vi "Demo - Log Analog and Digital Inputs to CSV File.vi"() -> ()   [LabVIEW 2021]
uses:
  TypeDefs/Enum - Machine State.ctl
  TypeDefs/TypeDef - Cluster of DAQiFi Device Properties.ctl
  TypeDefs/Enum - Connection Type.ctl
  <vilib>/Utility/file.llb/Write Delimited Spreadsheet (DBL).vi
  <vilib>/ErrorRing/Error Ring.xnode
panel:
  out "Digital Inputs":T1(graph)
  in  "Path - Saved CSV File":path=path "C:/Daqifi datafile.CSV"
  in  "Sampling Rate (Hz)":i32=1 min=1 max=1000 step=1
  out "Program Status":string
  in  "Stop":bool
  out "Analog Inputs":T2(graph)
  in  "DAQ IP Address or COM Port":string="192.168.1.1"
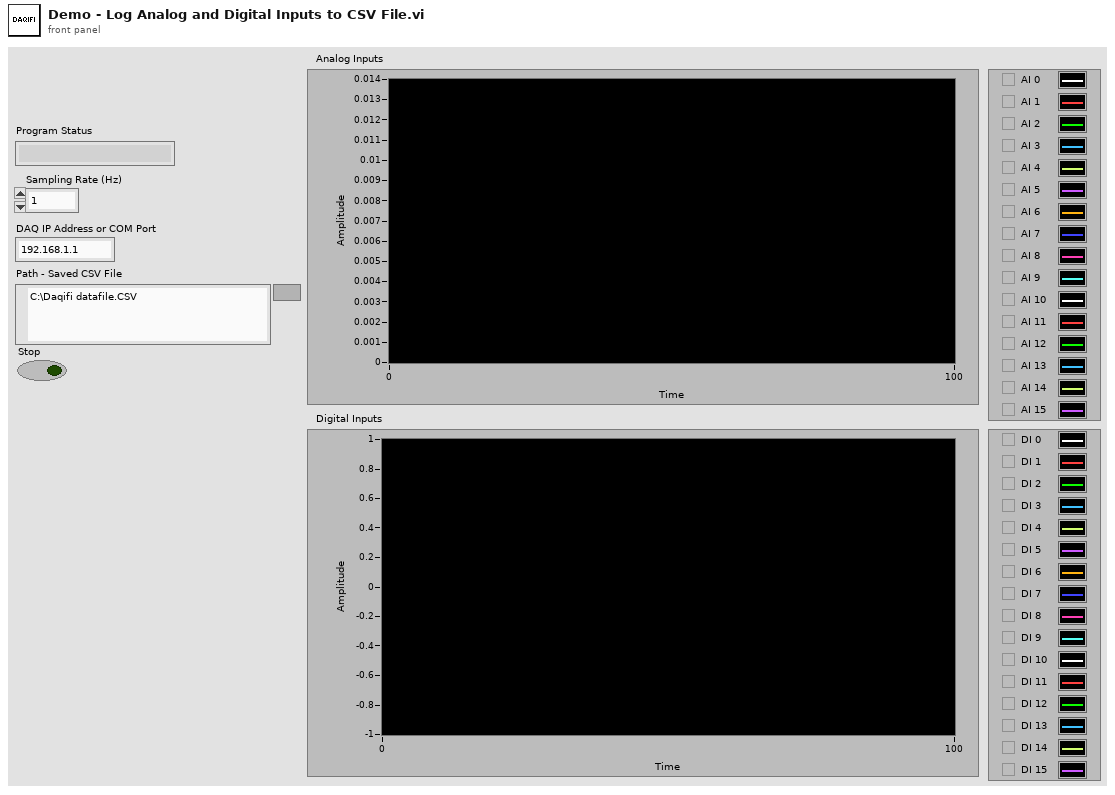
[diagram p1: front panel]
types:
  T1 = cluster{"[0]":dbl, "[1]":dbl, "[2]":dbl, "[3]":dbl, "[4]":dbl, "[5]":dbl, "[6]":dbl, "[7]":dbl, "[8]":dbl}
  T2 = cluster{"Array of Voltages (V)[0]":dbl, "Array of Voltages (V)[1]":dbl, "Array of Voltages (V)[2]":dbl, "Array of Voltages (V)[3]":dbl, "Array of Voltages (V)[4]":dbl, "Array of Voltages (V)[5]":dbl, "Array of Voltages (V)[6]":dbl, "Array of Voltages (V)[7]":dbl, "Array of Voltages (V)[8]":dbl}
  T3 = typedef "TypeDef - Cluster of DAQiFi Device Properties.ctl" = cluster{"IP Address":string, "MAC Address":string, "Serial Number":string, "Connection Type":T4, "Connected":bool, "TCP Network Connection":refnum<k5>, "USB Serial Connection":refnum<visa-resource-name>}
  T4 = typedef "Enum - Connection Type.ctl" = enum16{"USB", "TCP"}
  T5 = typedef "Enum - Machine State.ctl" = enum16{"Shutdown", "Save Data", "Start Streaming", "Initialize", "Read Streamed Data"}
  T6 = enum16{"open", "replace", "create", "open or create", "replace or create", "replace or create with confirmation"}
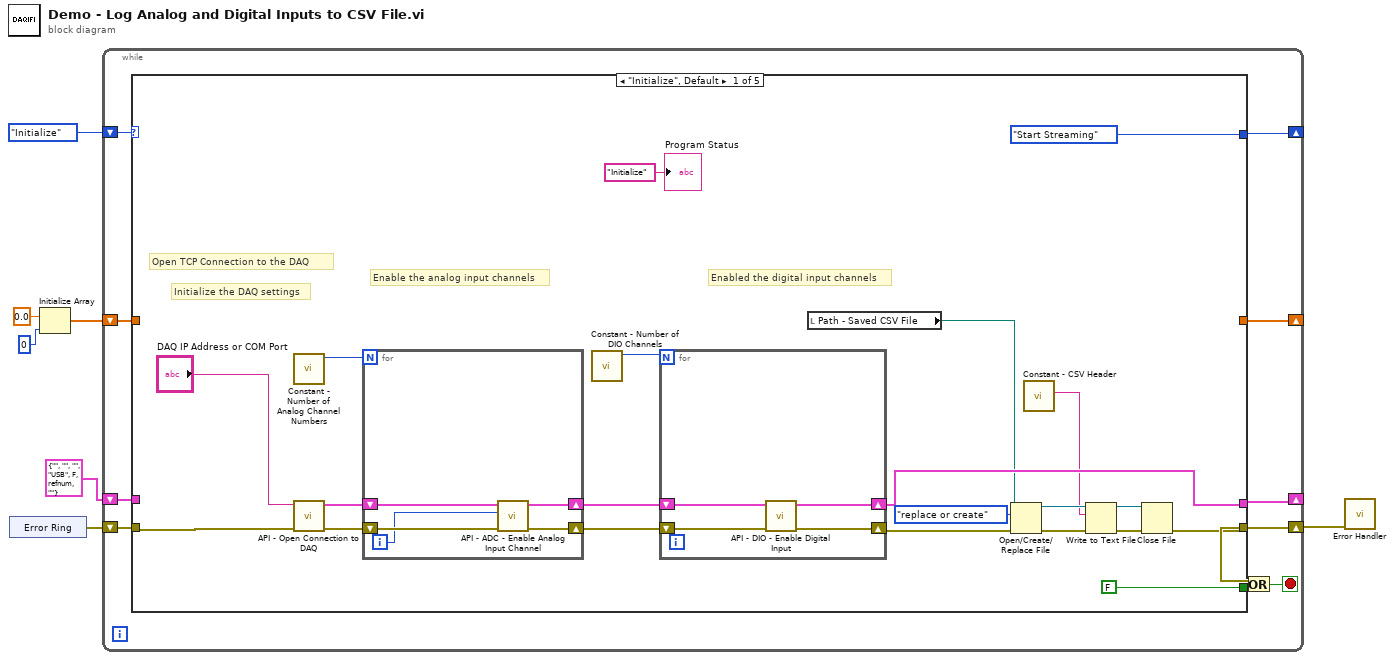
[diagram p0: block diagram]
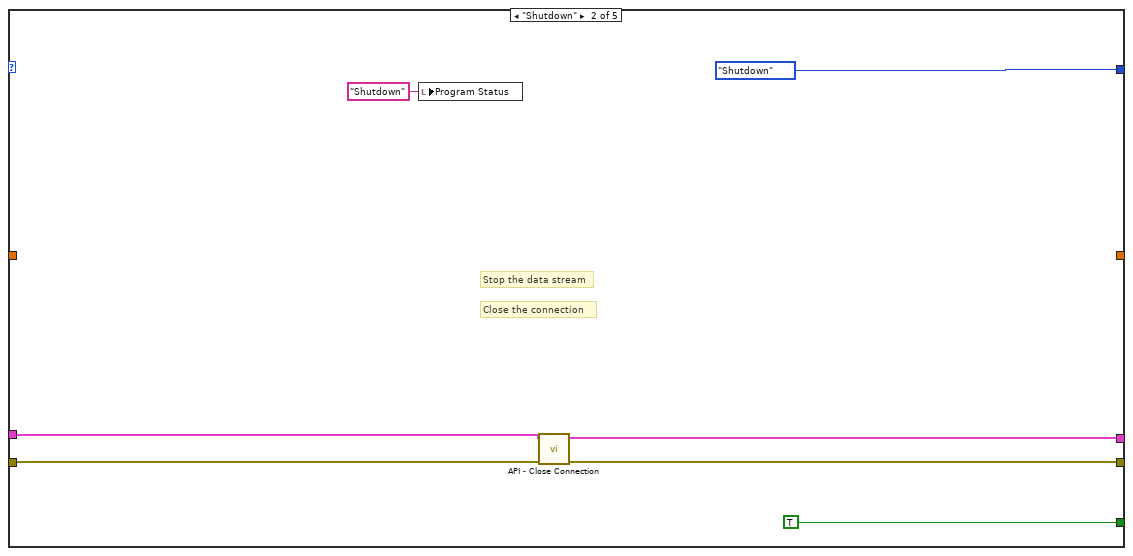
[diagram p2: hidden frame]
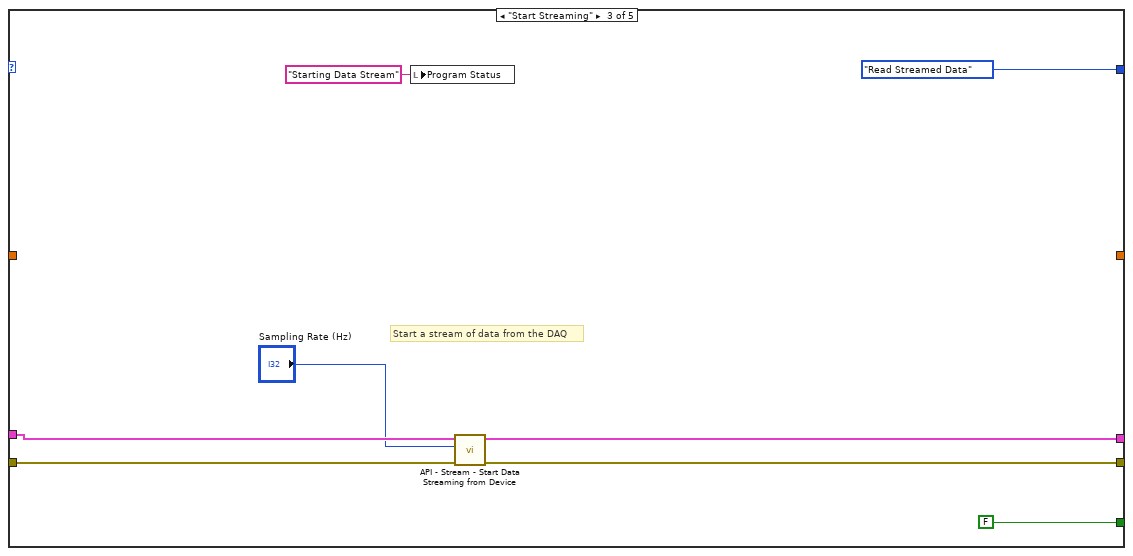
[diagram p3: hidden frame]
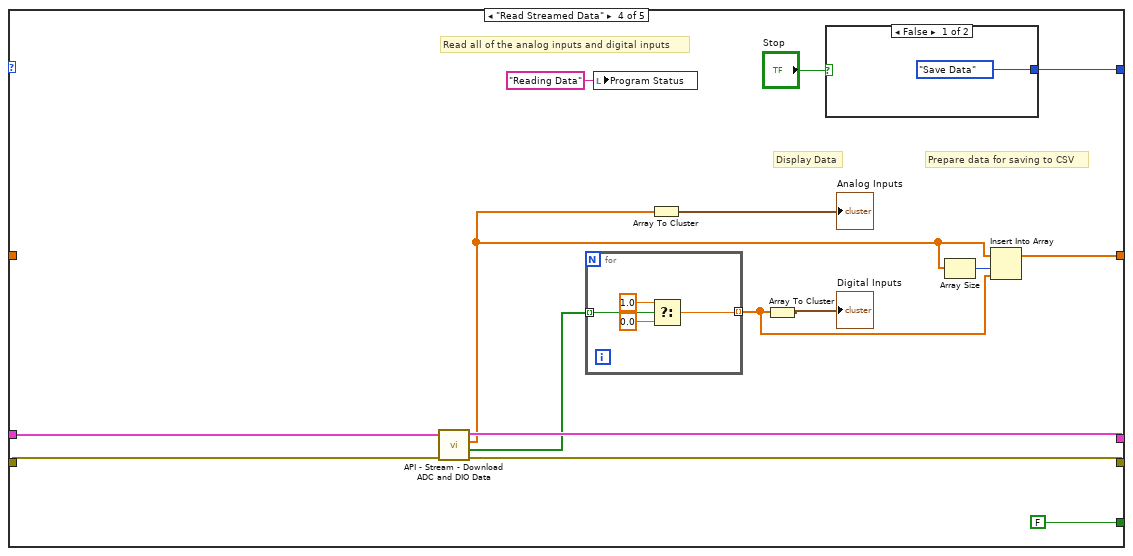
[diagram p4: hidden frame]
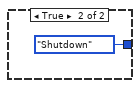
[diagram p5: hidden frame]
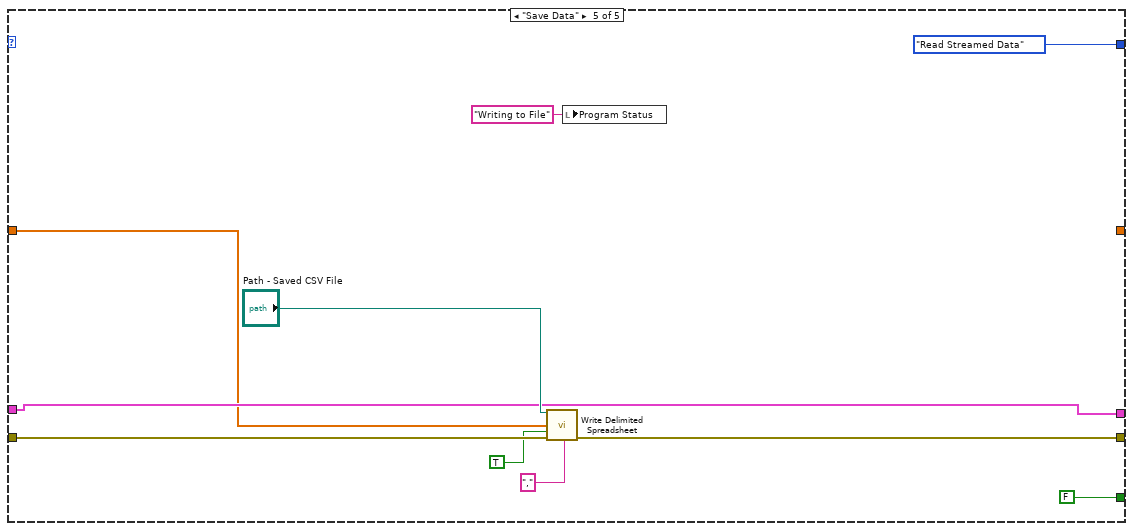
[diagram p6: hidden frame]
diagram:
  n1 = xnode "Error Ring"() -> ("error out"=w6:errorcluster)
  n2 = Initialize Array(0.0 ("element"), 0 ("dimension size")) -> (w2:dbl[])
  n3 = while {
    shift-right: [w11] -> w5
    shift-left: w6 -> [w16]
    shift-right: [w15] -> _
    shift-left: T3 {"IP Address"="", "MAC Address"="", "Serial Number"="", "Connection Type"=enum."USB", "Connected"=FALSE, "TCP Network Connection"=refnum, "USB Serial Connection"=""} ("DAQiFi Device Properties") -> [w13]
    shift-right: [w14] -> _
    shift-left: Enum_-_Machine_State."Initialize" -> [w17]
    shift-right: [w9] -> _
    shift-left: w2 -> [w8]
    stop <- w10 stop-if-true
    n4 = case shown="\"Initialize\", Default" w17 {
      tunnel: w16 -> [w33 w50 w56 w72 w92]
      tunnel: [w20 w49 w57 w71 w91] -> w11
      tunnel: [w27 w48 w58 w70 w87] -> w15
      tunnel: [Enum_-_Machine_State."Start Streaming" Enum_-_Machine_State."Shutdown" Enum_-_Machine_State."Read Streamed Data" w77 Enum_-_Machine_State."Read Streamed Data"] -> w14
      tunnel: [FALSE TRUE FALSE FALSE FALSE] -> w12
      tunnel: w13 -> [_ w51 w59 w73 w87]
      tunnel: [_ _ _ w67 _] -> w9
      tunnel: w8 -> [_ _ _ _ w86]
      frame "Initialize", Default {
        # "Enabled the digital input channels"
        # "Enable the analog input channels"
        # "Open TCP Connection to the DAQ"
        # "Initialize the DAQ settings"
        n5 = call "Constant - Number of Analog Channel Numbers.vi"() -> ("Maximum Channel"=w31:i32)  [unwired: 11 in]
        n6 = call "API - Open Connection to DAQ.vi"("error in"=w33, "DAQ Address (IP or COM)"="DAQ IP Address or COM Port") -> ("error out"=w32:errorcluster, "DAQiFi Device Properties"=w34:T3)  [unwired: 8 in]
        n7 = for {
          N: w31 -> [_]
          shift-right: [w47] -> w30
          shift-left: w34 -> [w45]
          shift-right: [w46] -> w29
          shift-left: w32 -> [w44]
          i -> [w43]
          n8 = call "API - ADC - Enable Analog Input Channel.vi"("error in (no error)"=w44, "Analog Input Channel Number"=w43, "DAQiFi Device Properties In"=w45) -> ("error out"=w46:errorcluster, "DAQiFi Device Properties Out"=w47:T3)  [unwired: 7 in]
        }
        n9 = call "Constant - Number of DIO Channels.vi"() -> ("Maximum Channel"=w28:i32)  [unwired: 11 in]
        n10 = for {
          N: w28 -> [_]
          shift-right: [w41] -> w27
          shift-left: w30 -> [w42]
          shift-right: [w39] -> w26
          shift-left: w29 -> [w40]
          n11 = call "API - DIO - Enable Digital Input.vi"("error in"=w40, "DAQiFi Device Properties In"=w42) -> ("error out"=w39:errorcluster, "DAQiFi Device Properties Out"=w41:T3)  [unwired: 8 in]
        }
        n12 = local read "Path - Saved CSV File"() -> (w23:path)
        n13 = Open/Create/Replace File(file path (use dialog)=w23, error in=w26, operation (0:open)=T6."replace or create") -> (refnum out=w24:refnum<file>, error out=w25:errorcluster)  [unwired: 3 in, 1 out]
        n14 = call "Constant - CSV Header.vi"() -> ("CSV Header"=w18:string)  [unwired: 11 in]
        n15 = Write to Text File(file (use dialog)=w24, text=w18, error in=w25) -> (refnum out=w19:refnum<file>, error out=w21:errorcluster)  [unwired: 1 in, 1 out]
        n16 = Close File(refnum=w19, error in=w21) -> (error out=w20:errorcluster)  [unwired: 1 out]
        "Program Status" <- "Initialize" ("Program Status")
      }
      frame "Shutdown" {
        # "Close the connection"
        # "Stop the data stream"
        n17 = local write "Program Status"("Shutdown" ("Program Status")) -> ()
        n18 = call "API - Close Connection.vi"("error in"=w50, "DAQiFi Device Properties In"=w51) -> ("error out"=w49:errorcluster, "DAQiFi Device Properties Out"=w48:T3)  [unwired: 8 in]
      }
      frame "Start Streaming" {
        # "Start a stream of data from the DAQ"
        n19 = local write "Program Status"("Starting Data Stream" ("Program Status")) -> ()
        n20 = call "API - Stream - Start Data Streaming from Device.vi"("error in"=w56, "Streaming Rate (Hz)"="Sampling Rate (Hz)", "DAQiFi Device Properties In"=w59) -> ("error out"=w57:errorcluster, "DAQiFi Device Properties Out"=w58:T3)  [unwired: 7 in]
      }
      frame "Read Streamed Data" {
        # "Prepare data for saving to CSV"
        # "Display Data"
        # "Read all of the analog inputs and digital inputs"
        n21 = call "API - Stream - Download ADC and DIO Data.vi"("error in"=w72, "DAQiFi Device Properties In"=w73) -> ("error out"=w71:errorcluster, "Digital Inputs"=w69:bool[], "Array of Voltages (V)"=w66:dbl[], "DAQiFi Device Properties Out"=w70:T3)  [unwired: 6 in]
        n22 = for {
          tunnel: w69 -> [w81] mode=indexing
          tunnel: [w78] -> w63 mode=indexing
          n23 = Select(t=1.0, s=w81, f=0.0) -> (s? t:f=w78:dbl)
        }
        n24 = local write "Program Status"("Reading Data" ("Program Status")) -> ()
        n25 = Array To Cluster(array=w66) -> (cluster=→"Analog Inputs":T2)
        n26 = Array To Cluster(array=w63) -> (cluster=→"Digital Inputs":T1)
        n27 = case shown="False" "Stop" {
          tunnel: [Enum_-_Machine_State."Save Data" Enum_-_Machine_State."Shutdown"] -> w77
          frame False {
          }
          frame True {
          }
        }
        n28 = Array Size(array=w66) -> (size(s)=w68:i32)
        n29 = Insert Into Array(array=w66, index=w68, new element=w63) -> (w67:dbl[])
      }
      frame "Save Data" {
        n30 = call-poly <vilib>:"Write Delimited Spreadsheet.vi"("file path (dialog if empty)"="Path - Saved CSV File", "1D data"=w86, "append to file? (new file:F)"=TRUE, "error in (no error)"=w92, "delimiter (\\t)"="," ("delimiter (\\t)")) -> ("error out"=w91:errorcluster)  [unwired: 9 in, 1 out]
        n31 = local write "Program Status"("Writing to File" ("Program Status")) -> ()
      }
    }
    n32 = Or(x=w11, y=w12) -> (x .or. y?=w10:bool)
  }
  n33 = call "Error Handler.vi"("error in"=w5) -> ()  [unwired: 10 in, 1 out]
